vi "VNA Driver Calibration Popup.vi"(8 "error in (no error)":errorcluster, 10 "RequestedCal":string="Manual Calibration of the E5071B VNA\r\n\r\nRequested Calibration:\r\n\tVNA CH1 - Response\r\n\tVNA CH2 - Response\r\n\tVNA CH3 - Response\r\n\tVNA CH4 - Response", 11 "Message (\"\")":string="The VNA stimulus parameters have been set, but the VNA requires a calibration.  Please perform the following steps:\n\n1)  Set the VNA to LOCAL mode operation by pressing the \"Local\" front panel key;\n2)  Set desired S-Parameter on the desired Channel;\n3)  Select the calibration menu by pressing the \"Cal\" front panel key;\n4)  Select an appropriate calibration procedure type by pressing the associated soft key;\n5)  Follow the instructions presented by the VNA to complete the selected calibration procedure. \n\nPress OK when the calibration procedure above is completed.") -> (0 "error out":errorcluster)   [LabVIEW 2011]
panel:
  in  "OK":bool
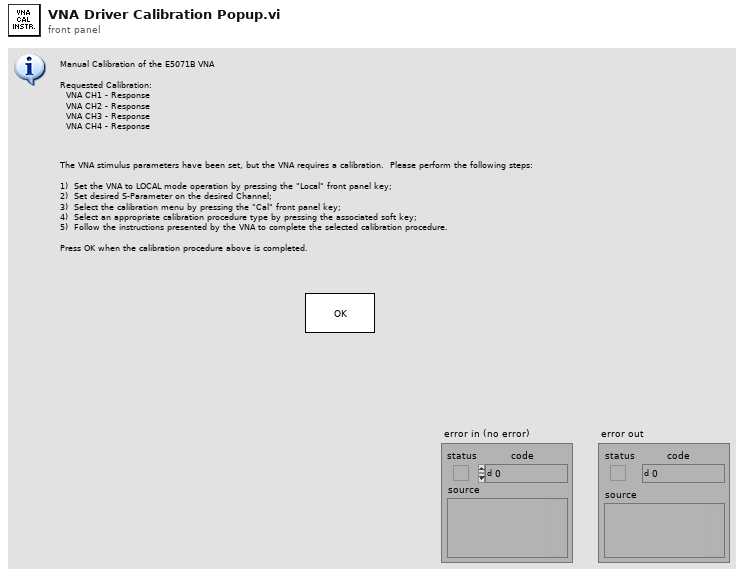
[diagram p1: front panel]
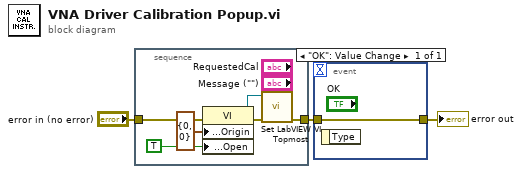
[diagram p0: block diagram]
diagram:
  n1 = stacked-sequence {
    tunnel: "error in (no error)" -> [w9]
    tunnel: [w6] -> w1
    frame #0 {
      n2 = property on="Property Node" class="VI"(error in=w9, "Front Panel Window:Origin"=cluster{"Horizontal":i16, "Vertical":i16} {"Horizontal"=0, "Vertical"=0}, "Front Panel Window:Open"=TRUE) -> (reference out=w5:refnum<vi>, error out=w7:errorcluster)  [unwired: 1 in]
      n3 = call "Set LabVIEW VI Topmost.vi"("error in (no error)"=w7, "VI Refnum (null)"=w5) -> ("error out"=w6:errorcluster)  [unwired: 7 in, 2 out]
    }
  }
  n4 = event shown="[0] \"OK\": Value Change" {
    selector: _ -> [_]
    dyn-events: _ -> [_]
    timeout: _ -> [_]
    tunnel: w1 -> [w10]
    tunnel: [w10] -> w3
    event "OK": Value Change {
      n5 = event-data() -> ()  [unwired: 2 out]
    }
  }
  "error out" <- w3
